vi "Load StandardWaveForm from XML.vi"() -> ()   [LabVIEW 2013]
uses:
  StandardWaveformWithName.ctl
  StandardWaveform.ctl
  <vilib>/xml/Load XML File.vi
  <vilib>/xml/Close Reference(Node).vi
  <vilib>/xml/NI_XML.lvlib
panel:
  out "node text":string
  in  "Cluster 2":T1={"Name"="", "Waveform"={"waveform type"=enum."sine", "amplitude"=1.0, "Time"=256.0}} caption="Cluster" {"Waveform"."amplitude" min=0.0 max=1.0 format="%.2f"}
  out "error IO":errorcluster
  out "parse errors":string
  in  "Path":path
  out "Cluster":T1={"Name"="", "Waveform"={"waveform type"=enum."sine", "amplitude"=1.0, "Time"=256.0}} {"Waveform"."amplitude" min=0.0 max=1.0 format="%.2f"}
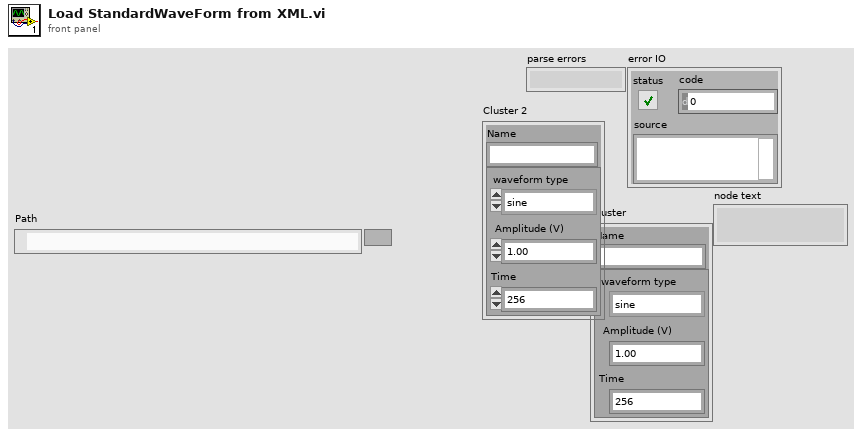
[diagram p1: front panel]
types:
  T1 = typedef "StandardWaveformWithName.ctl" = cluster{"Name":string, "Waveform":T2}
  T2 = typedef "StandardWaveform.ctl" = cluster{"waveform type":enum16{"sine", "cosine", "triangle", "square", "sawtooth", "increasing ramp", "decreasing ramp", "DC Value"}, "amplitude":dbl, "Time":dbl}
  T3 = enum16{"sine", "cosine", "triangle", "square", "sawtooth", "increasing ramp", "decreasing ramp", "DC Value"}
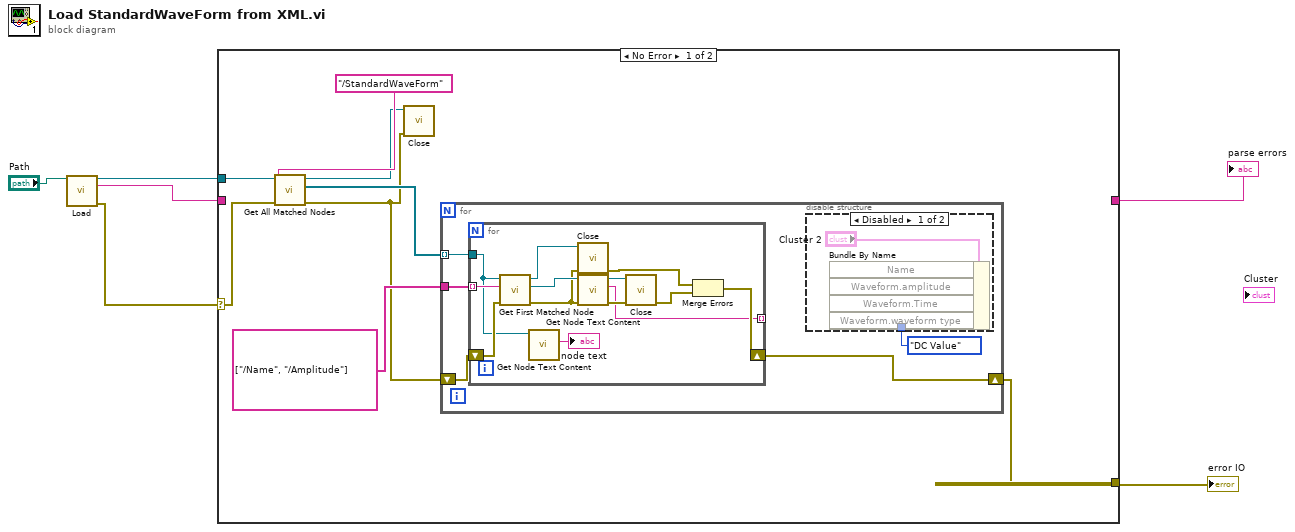
[diagram p0: block diagram]
diagram:
  n1 = call-poly <vilib>:"Load.vi"("path to XML document"="Path") -> ("DOM document out"=w5:refnum<k20>, "parse errors"=w3:string, "error out"=w4:errorcluster)  [unwired: 12 in]
  n2 = case shown="No Error" w4 {
    selector: w4 -> [w10 w35]
    tunnel: w5 -> [w14 _]
    tunnel: w3 -> [_ w36]
    tunnel: [_ w36] -> w2
    tunnel: [w9 w35] -> w1
    frame No Error {
      n3 = call <vilib>:"Get All Matched Nodes.vi"("error in (no error)"=w10, "XPath expression"="/StandardWaveForm", "node in"=w14) -> ("error out"=w7:errorcluster, "node result array"=w13:refnum<k20>[], "node out"=w11:refnum<k20>)  [unwired: 6 in]
      n4 = call-poly <vilib>:"Close.vi"("error in (no error)"=w7, "node"=w11) -> ()  [unwired: 7 in, 1 out]
      n5 = for {
        tunnel: w13 -> [w18] mode=indexing
        shift-right: [w17] -> w9
        shift-left: w7 -> [w19]
        tunnel: string[] ["/Name", "/Amplitude"] -> [w16]
        n6 = for {
          tunnel: w18 -> [w23]
          shift-right: [w26] -> w17
          shift-left: w19 -> [w32]
          tunnel: w16 -> [w25] mode=indexing
          tunnel: [w24] -> _ mode=indexing
          n7 = call <vilib>:"Get First Matched Node.vi"("error in (no error)"=w32, "XPath expression"=w25, "node in"=w23) -> ("error out"=w31:errorcluster, "node result"=w34:refnum<k20>, "node out"=w33:refnum<k20>)  [unwired: 6 in]
          n8 = call <vilib>:"Get Node Text Content.vi"("node in"=w23) -> ("node text"=→"node text":string)  [unwired: 8 in, 2 out]
          n9 = call-poly <vilib>:"Close.vi"("error in (no error)"=w31, "node"=w33) -> ("error out"=w27:errorcluster)  [unwired: 7 in]
          n10 = call <vilib>:"Get Node Text Content.vi"("error in (no error)"=w31, "node in"=w34) -> ("error out"=w29:errorcluster, "node text"=w24:string, "node out"=w30:refnum<k20>)  [unwired: 7 in]
          n11 = call-poly <vilib>:"Close.vi"("error in (no error)"=w29, "node"=w30) -> ("error out"=w28:errorcluster)  [unwired: 7 in]
          n12 = Merge Errors(w27, w28) -> (w26:errorcluster)
        }
        n13 = disable-structure shown="Disabled" {
          disable-tunnel: T3."DC Value" ("Waveform.waveform type") -> [w20 _]
          frame Disabled {
            n14 = Bundle By Name(cluster="Cluster 2", "Waveform.waveform type"=w20) -> ()  [unwired: 3 in, 1 out]
          }
          frame Enabled {
          }
        }
      }
    }
    frame Error {
    }
  }
  "parse errors" <- w2
  "error IO" <- w1
